vi "New Spritehandler.vi"(8 "error in (no error)":errorcluster) -> (0 "error out":errorcluster, 3 "SpriteHandler out":refnum<class "SpriteHandler.lvclass">)   [LabVIEW 2019, in "RT_Game.lvlib" / "SpriteHandler.lvclass"]
uses:
  SpriteHandler.lvclass
  RT_Sprite/RT_Sprite.lvclass
  SpriteHandler.lvclass/SpriteHandler.ctl
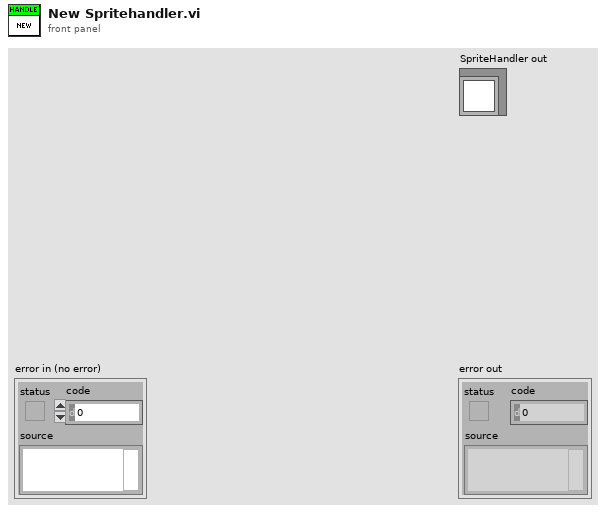
[diagram p1: front panel]
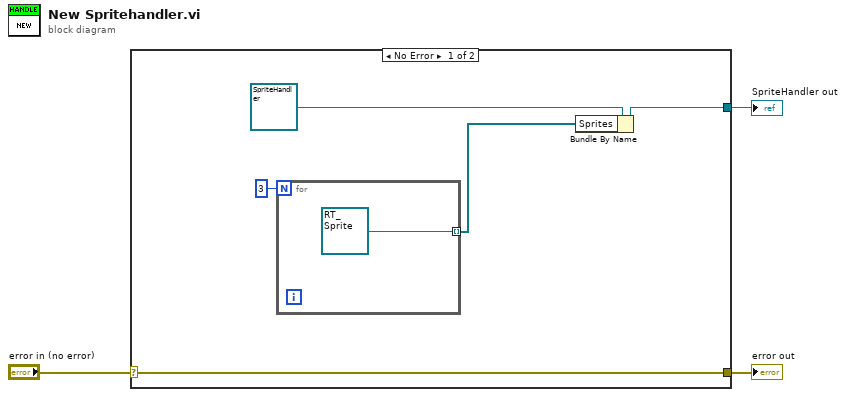
[diagram p0: block diagram]
diagram:
  n1 = case shown="No Error" "error in (no error)" {
    selector: "error in (no error)" -> [w8 w10]
    tunnel: [w8 w10] -> w2
    tunnel: [w6 _] -> w1
    frame No Error {
      n2 = for {
        N: 3 -> [_]
        tunnel: [refnum<class "RT_Sprite.lvclass"> refnum ("RT_Game.lvlib:RT_Sprite.lvclass")] -> w4 mode=indexing
      }
      n3 = Bundle By Name(cluster=refnum<class "SpriteHandler.lvclass"> refnum ("SpriteHandler out"), "Sprites"=w4) -> (w6:refnum<class "SpriteHandler.lvclass">)
    }
    frame Error {
    }
  }
  "error out" <- w2
  "SpriteHandler out" <- w1
